vi "Radar.vi"() -> ()   [LabVIEW 2012]
panel:
  in  "stop":bool
  out "2D Picture":picture
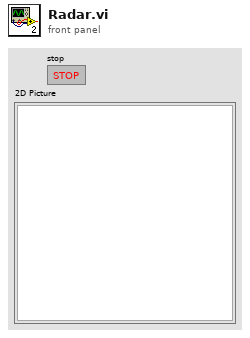
[diagram p1: front panel]
types:
  T1 = typedef "imagedata.ctl" = cluster{"image type":i32, "image depth":i32, "image":u8[], "mask":u8[], "colors":u32[], "Rectangle":cluster{"left":i16, "top":i16, "right":i16, "bottom":i16}}
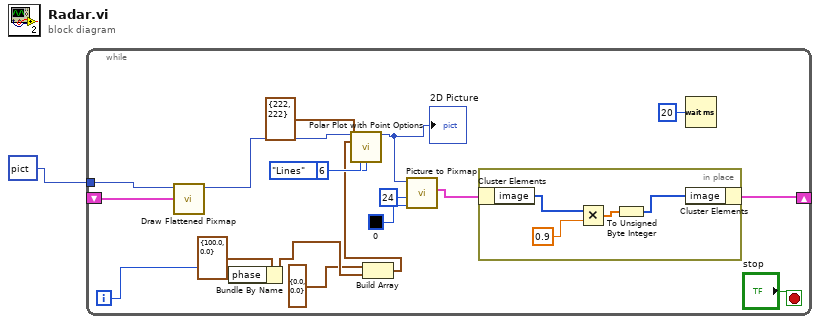
[diagram p0: block diagram]
diagram:
  n1 = while {
    shift-right: [w14] -> _
    shift-left: _ -> [w13]
    tunnel: picture data[5B] ("2D Picture") -> [w12]
    i -> [w7]
    stop <- "stop" stop-if-true
    n2 = call <vilib>:"Draw Flattened Pixmap.vi"("image data"=w13, "picture"=w12) -> ("new picture"=w19:picture)  [unwired: 7 in]
    n3 = Bundle By Name(cluster=cluster{"magnitude":dbl, "phase":dbl} {"magnitude"=100.0, "phase"=0.0}, "phase"=w7) -> (w9:cluster{"magnitude":dbl, "phase":dbl})
    n4 = Build Array(cluster{"magnitude":dbl, "phase":dbl} {"magnitude"=0.0, "phase"=0.0}, w9) -> (w3:cluster{"magnitude":dbl, "phase":dbl}[])
    n5 = call <vilib>:"Polar Plot with Point Options.vi"("picture"=w19, "data array [mag, phase (deg)]"=w3, "dimensions (w,h)"=cluster{"width":i16, "height":i16} {"width"=222, "height"=222}, "Lines/Points"=enum16{"Lines", "Points"}."Lines", "Size"=u16 6) -> ("new picture"=w18:picture)  [unwired: 10 in]
    "2D Picture" <- w18
    n6 = call <vilib>:"Picture to Pixmap.vi"("Background Color"=u32 0, "depth"=24, "picture"=w18) -> ("image data"=w15:T1)  [unwired: 7 in, 1 out]
    n7 = in-place {
      n8 = in-place-cluster #1(w15) -> ("image"=w23:u8[])
      n9 = Multiply(x=w23, y=0.9) -> (x*y=w21:dbl[])
      n10 = To Unsigned Byte Integer(number=w21) -> (unsigned 8bit integer=w20:u8[])
      n11 = in-place-cluster #1("image"=w20) -> (w14:T1)
    }
    n12 = Wait (ms)(milliseconds to wait=u32 20) -> ()  [unwired: 1 out]
  }
